vi "getI32Value.vi"(7 "Name":string, 8 "error in (no error)":errorcluster, 11 "tBSONDocument in":refnum<class "tBSONDocument.lvclass">) -> (0 "error out":errorcluster, 2 "Value":i32, 3 "tBSONDocument out":refnum<class "tBSONDocument.lvclass">)   [LabVIEW 2013, in "BSON.lvlib" / "tBSONDocument.lvclass"]
doc: "Retrieves an I32 from a BSON document."
uses:
  tBSONDocument.lvclass
  BSONElements/tBSON_I32/tBSON_I32.lvclass
  BSONElements/tBSON_I32/getValue.vi
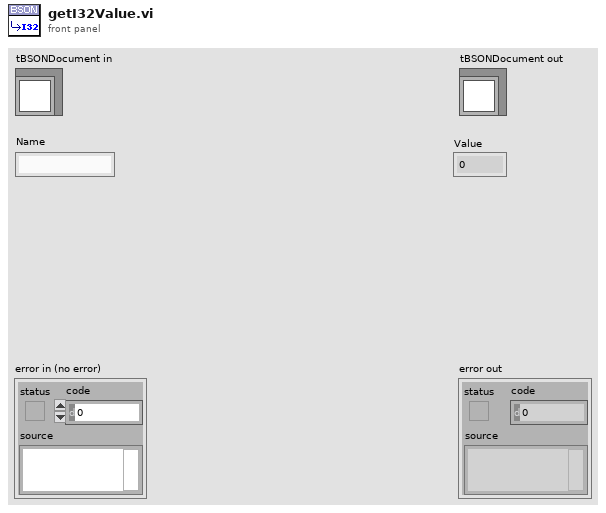
[diagram p1: front panel]
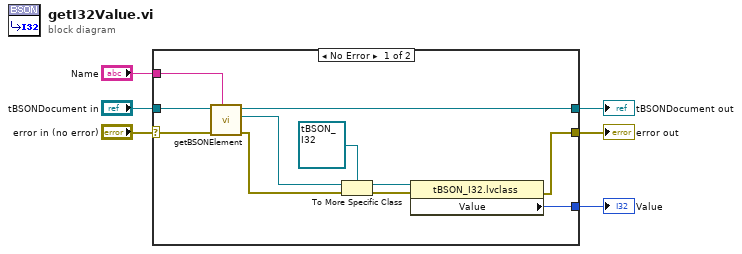
[diagram p0: block diagram]
diagram:
  n1 = case shown="No Error" "error in (no error)" {
    selector: "error in (no error)" -> [w16 w19]
    tunnel: [w9 w19] -> w5
    tunnel: [w10 w18] -> w3
    tunnel: "tBSONDocument in" -> [w17 w18]
    tunnel: "Name" -> [w7 _]
    tunnel: [w8 _] -> w1
    frame No Error {
      n2 = call "getBSONElement.vi"("Name"=w7, "error in (no error)"=w16, "tBSONDocument in"=w17) -> ("error out"=w12:errorcluster, "Element"=w13:refnum<class "tBSONElement.lvclass">, "tBSONDocument out"=w10:refnum<class "tBSONDocument.lvclass">)  [unwired: 6 in]
      n3 = To More Specific Class(target class=refnum<class "tBSON_I32.lvclass"> refnum ("BSON.lvlib:tBSON_I32.lvclass"), reference=w13, error in=w12) -> (specific class reference=w15:refnum<class "tBSON_I32.lvclass">, error out=w14:errorcluster)
      n4 = property class="tBSON_I32.lvclass"(reference=w15, error in=w14) -> (error out=w9:errorcluster, "Value"=w8:i32)  [unwired: 1 out]
    }
    frame Error {
    }
  }
  "error out" <- w5
  "tBSONDocument out" <- w3
  "Value" <- w1
